vi "mhk_Trap-Incremental_corrected_dA.vi"() -> ()   [LabVIEW 2010]
uses:
  <vilib>/Analysis/2dsp.llb/Integral Method.ctl
  <vilib>/Analysis/8numeric.llb/1D Numeric Integration.vi
  <vilib>/Analysis/NI_AALPro.lvlib
panel:
  out "function vector":dbl[](array[numeric])=[2.8782945992814364, 1.337771824193383, -0.16128951198299815, -1.4767801918167804, -2.4667815713080614, -3.0044534989569374, -2.99395137493301, -2.385636098463295, -1.1885234746810092, 0.5221888739878988, 2.6045033769083, 4.857386906851698, 7.037528698908553, 8.88453094782017, 10.152595929473714, 10.645366573647317, 10.249366470221279, 8.960729003050485, 6.8998545152511195, 4.309481854245292, 1.5334858840109356, -1.0235679572200387, -2.952746178318148, -3.9061068276209103, -3.6612758425870773, -2.1736373442356864, 0.3954037436251406, 3.6832916542675007, 7.168852767814431, 10.250435583666178, 12.35005725159535, 13.026864613200475, 12.078243166855195, 9.605643735343044, 6.025765582400926, 2.0163860261569853, -1.6010552584326068, -4.025181268566338, -4.654110846082377, -3.241123876892166, 0.013756605969474655]
  out "accumulated da vector":dbl[](array[numeric])=[0.0, 0.10540166058687049, 0.1348137183921301, 0.09386197579713564, -0.004727068280985416, -0.14150794503761038, -0.2914680668848591, -0.42595775371976674, -0.5153117430483743, -0.5319701080657021, -0.45380280179329713, -0.2672555446992972, 0.030117345444709065, 0.42816883661292715, 0.9040970085452743, 1.4240460711233, 1.946414397220015, 2.4266667840518092, 2.8231813720093495, 3.1034147812467596, 3.2494889747031652, 3.2622369228729378, 3.162829069484483, 2.9913577443360064, 2.8021731775808068, 2.656300347910238, 2.611844507894974, 2.71381189284229, 2.985115503394338, 3.4205977121813533, 3.9856100330628914, 4.620033079682787, 5.247660774184179, 5.789757946739135, 6.180543179682735, 6.381596969896682, 6.391980239089792, 6.251324325914818, 6.0343420230486, 5.836961154974237, 5.756276973201169]
  out "Integral X":dbl[](array[numeric])=[0.0, 0.10540166058687049, 0.1348137183921301, 0.09386197579713564, -0.004727068280985416, -0.14150794503761038, -0.2914680668848591, -0.42595775371976674, -0.5153117430483743, -0.5319701080657021, -0.45380280179329713, -0.2672555446992972, 0.030117345444709103, 0.4281688366129272, 0.9040970085452743, 1.4240460711233, 1.946414397220015, 2.4266667840518092, 2.8231813720093495, 3.1034147812467596, 3.2494889747031652, 3.2622369228729378, 3.162829069484483, 2.9913577443360064, 2.8021731775808068, 2.656300347910238, 2.611844507894974, 2.71381189284229, 2.985115503394338, 3.4205977121813533, 3.9856100330628914, 4.620033079682787, 5.247660774184179, 5.789757946739135, 6.180543179682735, 6.381596969896682, 6.391980239089792, 6.251324325914818, 6.0343420230486, 5.836961154974237, 5.756276973201169]
  out "raw da vector":dbl[](array[numeric])=[0.0, 0.10540166058687049, 0.029412057805259618, -0.04095174259499447, -0.09858904407812105, -0.13678087675662498, -0.14996012184724872, -0.13448968683490764, -0.08935398932860761, -0.01665836501732776, 0.07816730627240498, 0.18654725709399994, 0.29737289014400625, 0.3980514911682181, 0.47592817193234715, 0.5199490625780258, 0.522368326096715, 0.4802523868317941, 0.39651458795754013, 0.2802334092374103, 0.14607419345640568, 0.012747948169772422, -0.09940785338845468, -0.1714713251484765, -0.18918456675519968, -0.1458728296705691, -0.04445584001526365, 0.10196738494731604, 0.27130361055204827, 0.43548220878701527, 0.5650123208815382, 0.6344230466198957, 0.6276276945013918, 0.542097172554956, 0.39078523294359924, 0.20105379021394781, 0.010383269193109463, -0.1406559131749736, -0.21698230286621786, -0.19738086807436359, -0.0806841817730673]
  out "function\nvector\nsize":i32=41
  out "da\nvector\nsize":i32=41
  out "1D integration\nresult":dbl=5.75627697320117 format="%0.5f"
  out "Running Integral Graph":cluster{"Lower limit \"a\"":dbl, dbl, dbl[][]}(graph)={"Lower limit \"a\""=2.8, 0.05, [[0.0, 0.10540166058687049, 0.029412057805259618, -0.04095174259499447, -0.09858904407812105, -0.13678087675662498, -0.14996012184724872, -0.13448968683490764, -0.08935398932860761, -0.01665836501732776, 0.07816730627240498, 0.18654725709399994, 0.29737289014400625, 0.3980514911682181, 0.47592817193234715, 0.5199490625780258, 0.522368326096715, 0.4802523868317941, 0.39651458795754013, 0.2802334092374103, 0.14607419345640568, 0.012747948169772422, -0.09940785338845468, -0.1714713251484765, -0.18918456675519968, -0.1458728296705691, -0.04445584001526365, 0.10196738494731604, 0.27130361055204827, 0.43548220878701527, 0.5650123208815382, 0.6344230466198957, 0.6276276945013918, 0.542097172554956, 0.39078523294359924, 0.20105379021394781, 0.010383269193109463, -0.1406559131749736, -0.21698230286621786, -0.19738086807436359, -0.0806841817730673], [0.0, 0.10540166058687049, 0.1348137183921301, 0.09386197579713564, -0.004727068280985416, -0.14150794503761038, -0.2914680668848591, -0.42595775371976674, -0.5153117430483743, -0.5319701080657021, -0.45380280179329713, -0.2672555446992972, 0.030117345444709065, 0.42816883661292715, 0.9040970085452743, 1.4240460711233, 1.946414397220015, 2.4266667840518092, 2.8231813720093495, 3.1034147812467596, 3.2494889747031652, 3.2622369228729378, 3.162829069484483, 2.9913577443360064, 2.8021731775808068, 2.656300347910238, 2.611844507894974, 2.71381189284229, 2.985115503394338, 3.4205977121813533, 3.9856100330628914, 4.620033079682787, 5.247660774184179, 5.789757946739135, 6.180543179682735, 6.381596969896682, 6.391980239089792, 6.251324325914818, 6.0343420230486, 5.836961154974237, 5.756276973201169], [0.0, 0.10540166058687049, 0.1348137183921301, 0.09386197579713564, -0.004727068280985416, -0.14150794503761038, -0.2914680668848591, -0.42595775371976674, -0.5153117430483743, -0.5319701080657021, -0.45380280179329713, -0.2672555446992972, 0.030117345444709103, 0.4281688366129272, 0.9040970085452743, 1.4240460711233, 1.946414397220015, 2.4266667840518092, 2.8231813720093495, 3.1034147812467596, 3.2494889747031652, 3.2622369228729378, 3.162829069484483, 2.9913577443360064, 2.8021731775808068, 2.656300347910238, 2.611844507894974, 2.71381189284229, 2.985115503394338, 3.4205977121813533, 3.9856100330628914, 4.620033079682787, 5.247660774184179, 5.789757946739135, 6.180543179682735, 6.381596969896682, 6.391980239089792, 6.251324325914818, 6.0343420230486, 5.836961154974237, 5.756276973201169]]}
  in  "Plot BG Color":bool
  out "Approx. Integral \nover entire range\ndone incrementally":dbl=5.75627697320117
  out "Approx. Integral \nover entire range\ndone en masse":dbl=5.75627697320117
  out "Function Graph":cluster{"Lower limit \"a\"":dbl, dbl, dbl[]}(graph)={"Lower limit \"a\""=2.8, 0.05, [2.8782945992814364, 1.337771824193383, -0.16128951198299815, -1.4767801918167804, -2.4667815713080614, -3.0044534989569374, -2.99395137493301, -2.385636098463295, -1.1885234746810092, 0.5221888739878988, 2.6045033769083, 4.857386906851698, 7.037528698908553, 8.88453094782017, 10.152595929473714, 10.645366573647317, 10.249366470221279, 8.960729003050485, 6.8998545152511195, 4.309481854245292, 1.5334858840109356, -1.0235679572200387, -2.952746178318148, -3.9061068276209103, -3.6612758425870773, -2.1736373442356864, 0.3954037436251406, 3.6832916542675007, 7.168852767814431, 10.250435583666178, 12.35005725159535, 13.026864613200475, 12.078243166855195, 9.605643735343044, 6.025765582400926, 2.0163860261569853, -1.6010552584326068, -4.025181268566338, -4.654110846082377, -3.241123876892166, 0.013756605969474655]}
  in  "Divisions \"N\"":dbl=40.0
  in  "Upper limit \"b\"":dbl=4.8
  in  "Lower limit \"a\"":dbl=2.8
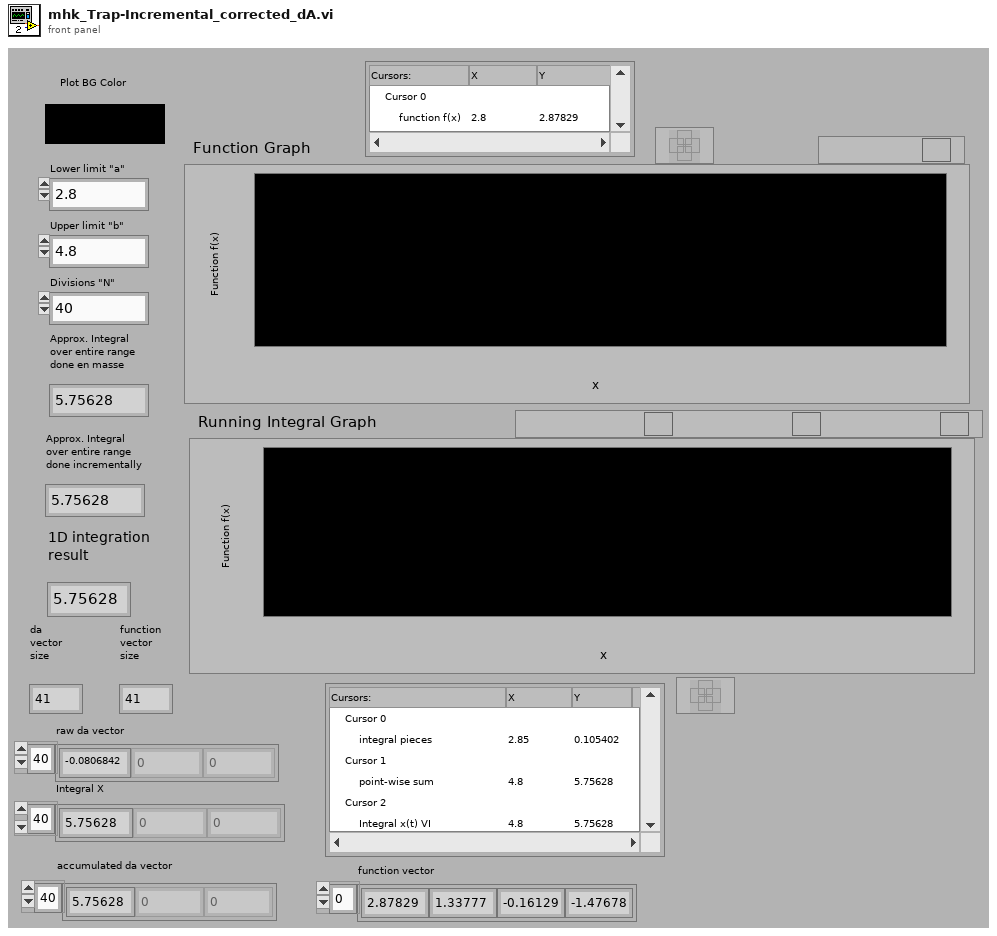
[diagram p1: front panel]
types:
  T1 = typedef "NI_AALPro.lvlib/Integral Method.ctl" = i32
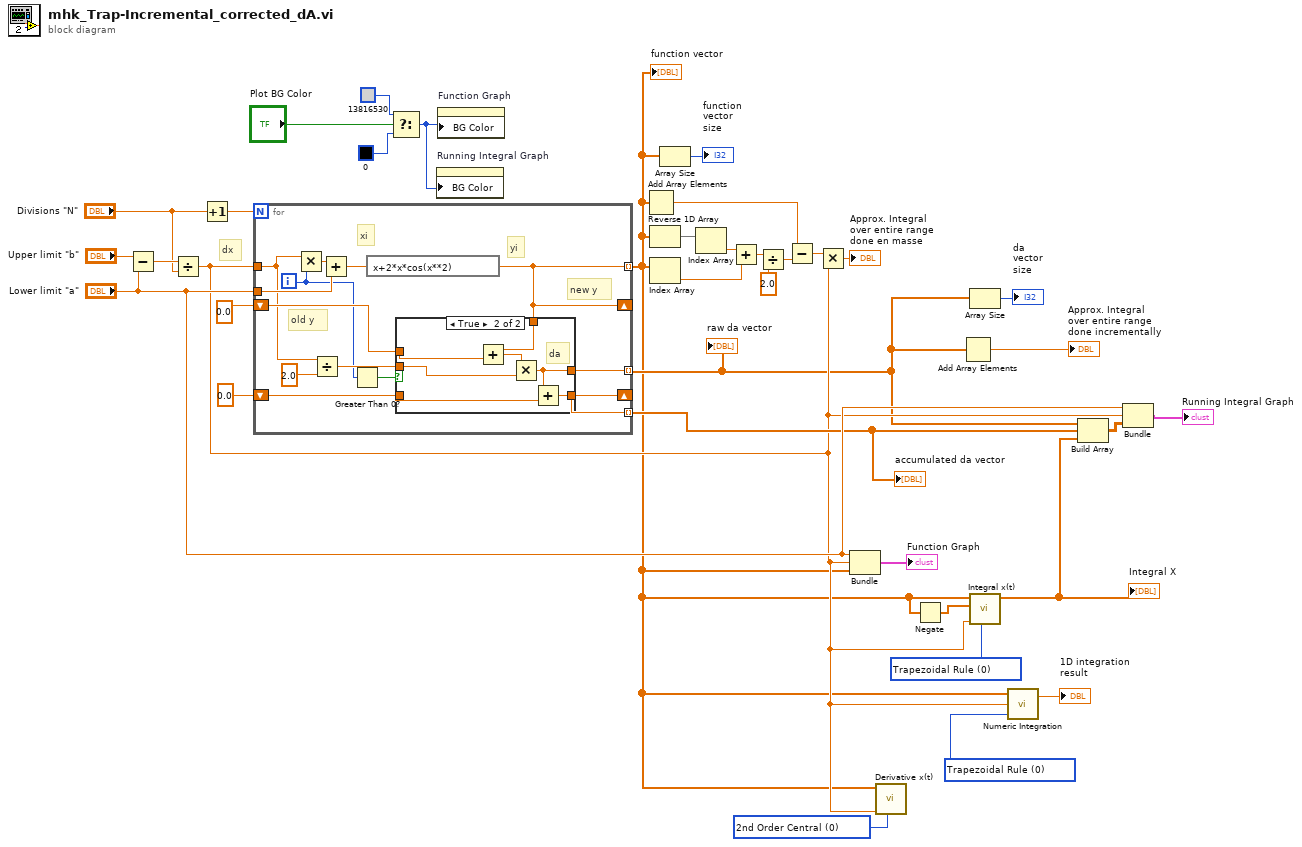
[diagram p0: block diagram]
diagram:
  w10 = u16 0 items=["2nd Order Central", "4th Order Central", "Forward", "Backward"] ("method")
  w12 = T1 0 items=["Trapezoidal Rule", "Simpson's Rule", "Simpson's 3/8 Rule", "Bode Rule"] ("integration method")
  w14 = T1 0 items=["Trapezoidal Rule", "Simpson's Rule", "Simpson's 3/8 Rule", "Bode Rule"] ("integration method")
  # "dx"
  n1 = Subtract(x="Upper limit \"b\"", y="Lower limit \"a\"") -> (x-y=w35:dbl)
  n2 = Divide(x=w35, y="Divisions \"N\"") -> (x/y=w11:dbl)
  n3 = Increment(x="Divisions \"N\"") -> (x+1=w34:dbl)
  n4 = for {
    N: w34 -> [_]
    tunnel: w11 -> [w38]
    tunnel: "Lower limit \"a\"" -> [w48]
    tunnel: [w46] -> w3 mode=indexing
    shift-right: [w46] -> _
    shift-left: 0.0 -> [w45]
    tunnel: [w42] -> w4 mode=indexing
    shift-right: [w40] -> _
    shift-left: 0.0 -> [w41]
    tunnel: [w40] -> w16 mode=indexing
    i -> [w37]
    # "new y"
    # "old y"
    # "yi"
    # "xi"
    n5 = Multiply(x=w38, y=w37) -> (x*y=w49:dbl)
    n6 = Divide(x=w38, y=2.0) -> (x/y=w43:dbl)
    n7 = Add(x=w49, y=w48) -> (x+y=w47:dbl)
    n8 = Greater Than 0?(x=w37) -> (x > 0?=w39:bool)
    n9 = expression code="x+2*x*cos(x**2)"(w47) -> (w46:dbl)
    n10 = case shown="True" w39 {
      tunnel: w46 -> [_ w57]
      tunnel: w45 -> [_ w56]
      tunnel: w43 -> [_ w54]
      tunnel: [w50 w53] -> w42
      tunnel: w41 -> [w50 w52]
      tunnel: [w50 w51] -> w40
      frame False {
      }
      frame True {
        # "da"
        n11 = Add(x=w57, y=w56) -> (x+y=w55:dbl)
        n12 = Multiply(x=w55, y=w54) -> (x*y=w53:dbl)
        n13 = Add(x=w53, y=w52) -> (x+y=w51:dbl)
      }
    }
  }
  "raw da vector" <- w4
  "accumulated da vector" <- w16
  "function vector" <- w3
  n14 = Select(t=u32 13816530, s="Plot BG Color", f=u32 0) -> (s? t:f=w17:u32)
  n15 = property on="Running Integral Graph" class="WFGraph (strict)"("BG Color"=w17) -> ()  [unwired: 2 in, 2 out]
  n16 = property on="Function Graph" class="WFGraph (strict)"("BG Color"=w17) -> ()  [unwired: 2 in, 2 out]
  n17 = Add Array Elements(numeric array=w3) -> (sum=w26:dbl)
  n18 = Reverse 1D Array(array=w3) -> (reversed array=w32:dbl[])
  n19 = Index Array(array=w3) -> (element=w30:dbl)  [unwired: 1 in]
  n20 = Array Size(array=w3) -> (size(s)=→"function\nvector\nsize":i32)
  n21 = Index Array(array=w32) -> (element=w31:dbl)  [unwired: 1 in]
  n22 = Add(x=w31, y=w30) -> (x+y=w29:dbl)
  n23 = Divide(x=w29, y=2.0) -> (x/y=w27:dbl)
  n24 = Subtract(x=w26, y=w27) -> (x-y=w25:dbl)
  n25 = Multiply(x=w25, y=w11) -> (x*y=→"Approx. Integral \nover entire range\ndone en masse":dbl)
  n26 = Bundle("Lower limit \"a\""="Lower limit \"a\"", w11, w3) -> (→"Function Graph":cluster{"Lower limit \"a\"":dbl, dbl, dbl[]})  [unwired: 1 in]
  n27 = call <vilib>:"Derivative x(t).vi"("method"=w10, "dt"=w11, "X"=w3) -> ()  [unwired: 7 in, 2 out]
  n28 = Negate(x=w3) -> (-x=w2:dbl[])
  n29 = Add Array Elements(numeric array=w4) -> (sum=→"Approx. Integral \nover entire range\ndone incrementally":dbl)
  n30 = Array Size(array=w4) -> (size(s)=→"da\nvector\nsize":i32)
  n31 = call <vilib>:"Integral x(t).vi"("integration method"=w12, "dt"=w11, "Initial Condition"=w2, "X"=w3) -> ("Integral X"=w6:dbl[])  [unwired: 6 in, 1 out]
  "Integral X" <- w6
  n32 = call-poly <vilib>:"Numeric Integration.vi"("integration method"=w14, "dt"=w11, "Input Array"=w3) -> ("result"=→"1D integration\nresult":dbl)  [unwired: 1 out]
  n33 = Build Array(w4, w16, w6) -> (w15:dbl[][])
  n34 = Bundle("Lower limit \"a\""="Lower limit \"a\"", w11, w15) -> (→"Running Integral Graph":cluster{"Lower limit \"a\"":dbl, dbl, dbl[][]})  [unwired: 1 in]
